vi "3.2.2-GPS.vi"(1 "stop":bool, 2 "VISA resource name":refnum<visa-resource-name>="ASRL1::INSTR") -> (0 "Current GPS Data":T1 {"Longitude (dd.mmmmmm)" format="%#.6g"; "Lattitude (dd.mmmmmm)" format="%#.6g"})   [LabVIEW 2010]
uses:
  4-High Neurons/Current GPS Data.ctl
  3.0-Global.vi
panel:
  out "GPS Data":T2 {"Course over ground (degrees)" format="%#.6g"; "Speed over ground (knots)" format="%#.6g"; "Magnetic Variation (degrees)" format="%#.6g"; "Longitude (dd.mmmmmm)" format="%#.6g"; "Lattitude (dd.mmmmmm)" format="%#.6g"}
  out "XY Graph":cluster{"Y":dbl[], "Y":dbl[]}[](graph)
  out "Course over ground (degrees)":dbl(knob) scale=0.0..360.0
  out "Speed over ground (knots)":dbl(knob) scale=0.0..5.0
  out "GPS Data Valid?":bool
  out "error out":errorcluster
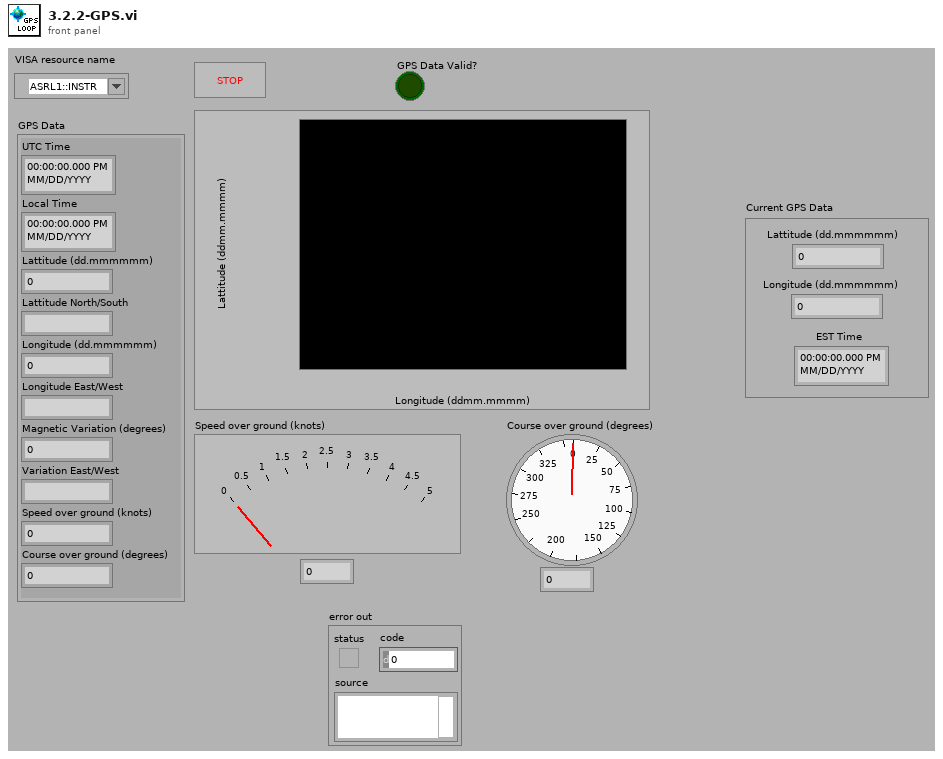
[diagram p1: front panel]
types:
  T1 = typedef "Current GPS Data.ctl" = cluster{"Lattitude (dd.mmmmmm)":ext, "Longitude (dd.mmmmmm)":ext, "EST Time":timestamp}
  T2 = cluster{"UTC Time":timestamp, "Local Time":timestamp, "Lattitude (dd.mmmmmm)":dbl, "Lattitude North/South":string, "Longitude (dd.mmmmmm)":dbl, "Longitude East/West":string, "Magnetic Variation (degrees)":dbl, "Variation East/West":string, "Speed over ground (knots)":dbl, "Course over ground (degrees)":dbl}
  T3 = cluster{"UTC Time":timestamp, "Local Time":timestamp, "Lattitude (ddmm.mmmm)":dbl, "Lattitude North/South":string, "Longitude (ddmm.mmmm)":dbl, "Longitude East/West":string, "Magnetic Variation (degrees)":dbl, "Variation East/West":string, "Speed over ground (knots)":dbl, "Course over ground (degrees)":dbl}
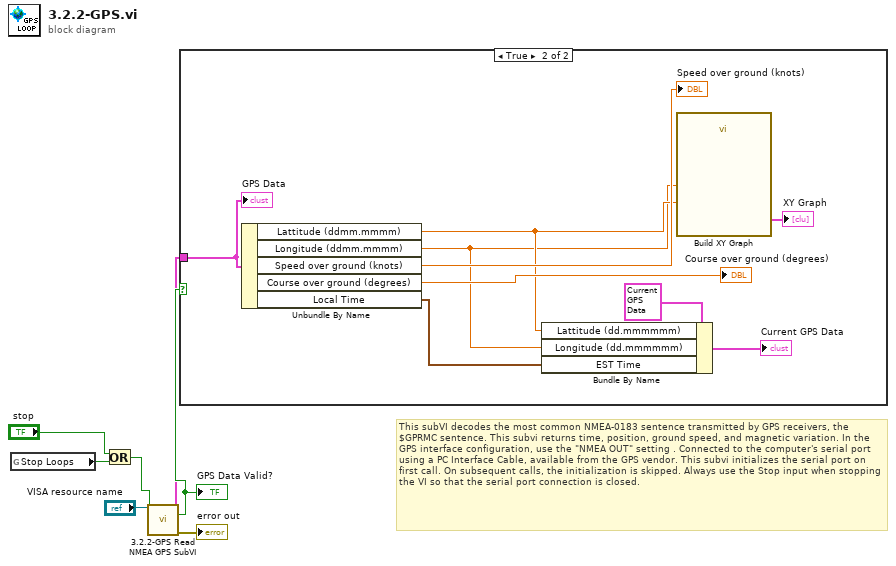
[diagram p0: block diagram]
diagram:
  # "This subVI decodes the most common NMEA-0183 sentence transmitted by GPS receivers, the $GPRMC sentence. This subvi returns time, position, ground speed, and magnetic variation. In the GPS interface configuration, use the \"NMEA OUT\" setting . Connected to the computer's serial port using a PC Interface Cable, available from the GPS vendor. This subvi initializes the serial port on first call. On subsequent calls, the initialization is skipped. Always use the Stop input when stopping the VI so that the serial port connection is closed."
  n1 = global read "3.0-Global.vi" "Stop Loops"() -> (w3:bool)
  n2 = Or(x="stop", y=w3) -> (x .or. y?=w2:bool)
  n3 = call "3.2.2-GPS Read NMEA GPS SubVI.vi"("VISA resource name"="VISA resource name", "stop"=w2) -> ("GPS Data"=w6:T3, "GPS Data Valid?"=w7:bool, "error out"=→"error out":errorcluster)  [unwired: 10 in, 1 out]
  "GPS Data Valid?" <- w7
  n4 = case shown="True" w7 {
    tunnel: w6 -> [_ w16]
    frame False {
    }
    frame True {
      n5 = Unbundle By Name(w16) -> ("Lattitude (ddmm.mmmm)"=w11:dbl, "Longitude (ddmm.mmmm)"=w10:dbl, "Speed over ground (knots)"=→"Speed over ground (knots)":dbl, "Course over ground (degrees)"=→"Course over ground (degrees)":dbl, "Local Time"=w9:timestamp)
      n6 = Bundle By Name(cluster=T1 {"Lattitude (dd.mmmmmm)"=42.1761676, "Longitude (dd.mmmmmm)"=71.1586789, "EST Time"=timestamp(3386095336 s since 1904-01-01)} ("GPS Data 2"), "Lattitude (dd.mmmmmm)"=w11, "Longitude (dd.mmmmmm)"=w10, "EST Time"=w9) -> (→"Current GPS Data":T1)
      n7 = call "Build XY Graph"("Y Input"=w11, "X Input"=w10) -> ("XY Graph"=→"XY Graph":cluster{"Y":dbl[], "Y":dbl[]}[])  [unwired: 8 in, 1 out]
      "GPS Data" <- w16
    }
  }
